vi "SetSTringValue by Ref.vi"(8 "错误输入（无错误）":errorcluster, 10 "字符串":string, 11 "String输入":refnum<vi>) -> ()   [LabVIEW 2017]
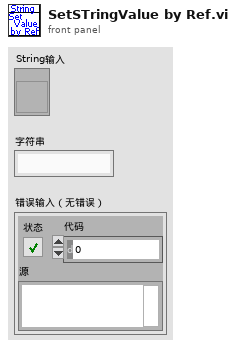
[diagram p1: front panel]
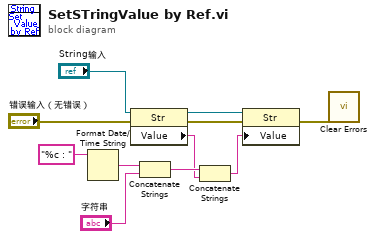
[diagram p0: block diagram]
diagram:
  n1 = Format Date/Time String(time format string (%c)="%c : " ("时间格式字符串(%c)")) -> (date/time string=w10:string)  [unwired: 2 in]
  n2 = property class="Str"(reference="String输入", error in="错误输入（无错误）") -> (reference out=w7:refnum<vi>, error out=w5:errorcluster, "Value"=w2:string)
  n3 = Concatenate Strings(w10, "字符串") -> (w3:string)
  n4 = Concatenate Strings(w3, w2) -> (w6:string)
  n5 = property class="Str"(reference=w7, error in=w5, "Value"=w6) -> (error out=w1:errorcluster)  [unwired: 1 out]
  n6 = call <vilib>:"Clear Errors.vi"("error in (no error)"=w1) -> ()  [unwired: 5 in, 2 out]
